vi "13-ATC예문.vi"() -> ()   [LabVIEW 2014]
doc: "ATC app"
uses:
  <vilib>/Utility/sysdir.llb/System Directory Type.ctl
panel:
  in  "정규식 3":string
  out "ip address":string="ip address 를 불러옵니다."
  in  "정규식":string
  in  "정규식 2":string
  out "연결된 문자열":string
  in  "탭 컨트롤":T1(tab)
  in  "메모":string="필요한 메모를 할수 있습니다. "
  in  "SID&RadarVector. 2":string="SID&RadarVector. "
  in  "인사말":string="인사말"
  in  "관제기관":string="관제기관"
  in  "콜사인":string="콜사인\n콜사인\n콜사인"
  in  "도착공항":string="도착공항"
  in  "SID&RadarVector":string="SID&RadarVector"
  in  "비행고도":string="비행고도"
  in  "인사말2":string="인사말"
  in  "콜사인2":string="콜사인"
  in  "콜사인3":string="콜사인"
  in  "콜사인4":string="콜사인"
  in  "콜사인5":string="콜사인"
  in  "콜사인6":string="콜사인"
  in  "도착공항2":string="도착공항"
  in  "제한고도":string="제한고도"
  in  "비행고도2":string="비행고도"
  in  "D접속주파수":string="접속주파수"
  in  "스콱번호":string="스콱번호"
  in  "도착공항3":string="도착공항"
  in  "SID&RadarVector. 3":string="SID&RadarVector. "
  in  "제한고도2":string="제한고도"
  in  "비행고도3":string="비행고도"
  in  "D접속주파수2":string="접속주파수"
  in  "스콱번호2":string="스쾃번호"
  in  "콜사인7":string="콜사인"
  in  "콜사인8":string="콜사인"
  in  "관제기관":string="관제기관"
  in  "G접속주파수2":string="접속주파수"
  in  "관제기관":string="관제기관"
  in  "G접속주파수":string="접속주파수"
  in  "콜사인9":string="콜사인"
  in  "정보1":bool
  in  "메모2":string="필요한 메모를 할수 있습니다. "
  in  "관제기관":string="관제기관"
  in  "콜사인24":string="콜사인"
  in  "T접속주파수2":string="접속주파수"
  in  "T접속주파수":string="접속주파수"
  in  "관제기관":string="관제기관"
  in  "콜사인23":string="콜사인"
  in  "활주로9":string="활주로"
  in  "관제기관":string="관제기관"
  in  "콜사인22":string="콜사인"
  in  "콜사인21":string="콜사인"
  in  "콜사인20":string="콜사인"
  in  "콜사인19":string="콜사인"
  in  "활주로8":string="활주로"
  in  "활주로7":string="활주로"
  in  "콜사인17":string="콜사인"
  in  "활주로6":string="활주로"
  in  "콜사인18":string="콜사인"
  in  "관제기관":string="관제기관"
  in  "then2":string="than"
  in  "활주로5":string="활주로"
  in  "콜사인16":string="콜사인"
  in  "then":string="than"
  in  "활주로4":string="활주로"
  in  "콜사인15":string="콜사인"
  in  "활주로3":string="활주로"
  in  "관제기관":string="관제기관"
  in  "콜사인14":string="콜사인"
  in  "콜사인13":string="콜사인"
  in  "현재기압2":string="현재기압"
  in  "출발공항":string="출발공항"
  in  "활주로2":string="활주로"
  in  "현재기압":string="현재기압"
  in  "출발공항":string="출발공항"
  in  "활주로1":string="활주로"
  in  "콜사인12":string="콜사인"
  in  "콜사인11":string="콜사인"
  in  "관제기관":string="관제기관"
  in  "인사3":string="인사"
  in  "정보2":bool
  in  "메모3":string="필요한 메모를 할수 있습니다. "
  in  "인사4":string="인사"
  in  "콜사인25":string="콜사인"
  in  "활주로10":string="활주로"
  in  "콜사인26":string="콜사인"
  in  "바람방향":string="바람방향"
  in  "풍속":string="풍속"
  in  "콜사인27":string="콜사인"
  in  "바람방향2":string="바람방향"
  in  "풍속2":string="풍속"
  in  "활주로11":string="활주로"
  in  "콜사인28":string="콜사인"
  in  "활주로13":string="활주로"
  in  "콜사인29":string="콜사인"
  in  "활주로12":string="활주로"
  in  "콜사인30":string="콜사인"
  in  "활주로14":string="활주로"
  in  "콜사인31":string="콜사인"
  in  "활주로15":string="활주로"
  in  "관제기관":string="관제기관"
  in  "콜사인32":string="콜사인"
  in  "현재고도":string="현재고도"
  in  "허가고도":string="허가고도"
  in  "콜사인33":string="콜사인"
  in  "접속주파수":string="접속주파수"
  in  "콜사인34":string="콜사인"
  in  "접속주파수2":string="접속주파수"
  in  "정보3":bool
  in  "메모 4":string="필요한 메모를 할수 있습니다. "
  in  "인사5":string="인사"
  in  "관제기관":string="관제기관"
  in  "콜사인35":string="콜사인"
  in  "거리":string="거리"
  in  "지점":string="지점"
  in  "현재고도A":string="현재고도"
  in  "허가고도3":string="허가고도"
  in  "콜사인36":string="콜사인"
  in  "관제기관":string="관제기관"
  in  "허가고도4":string="허가고도"
  in  "허가고도5":string="허가고도"
  in  "콜사인37":string="콜사인"
  in  "콜사인38":string="콜사인"
  in  "허가고도6":string="허가고도"
  in  "허가고도7":string="허가고도"
  in  "콜사인39":string="콜사인"
  in  "콜사인40":string="콜사인"
  in  "거리2":string="거리"
  in  "지점2":string="지점"
  in  "관제기관":string="관제기관"
  in  "A접속주파수":string="접속주파수"
  in  "관제기관":string="관제기관"
  in  "A접속주파수2":string="접속주파수"
  in  "콜사인41":string="콜사인"
  in  "정보4":bool
  in  "콜사인42":string="콜사인"
  in  "관제기관":string="관제기관"
  in  "A접속주파수":string="접속주파수"
  in  "콜사인45":string="콜사인"
  in  "관제기관":string="관제기관"
  in  "A접속주파수2":string="접속주파수"
  in  "관제기관":string="관제기관"
  in  "콜사인46":string="콜사인"
  in  "날시정보":string="날시정보"
  in  "고도":string="고도"
  in  "콜사인47":string="콜사인"
  in  "관제기관":string="관제기관"
  in  "L활주로":string="활주로"
  in  "도착공항4":string="도착공항"
  in  "현재기압":string="현재기압"
  in  "콜사인48":string="콜사인"
  in  "관제기관5":string="관제기관"
  in  "L활주로":string="활주로"
  in  "도착공항5":string="도착공항"
  in  "현재기압":string="현재기압"
  in  "콜사인49":string="콜사인"
  in  "고도":string="고도"
  in  "콜사인50":string="콜사인"
  in  "고도":string="고도"
  in  "콜사인51":string="콜사인"
  in  "고도":string="고도"
  in  "고도":string="고도"
  in  "콜사인52":string="콜사인"
  in  "콜사인53":string="콜사인"
  in  "관제기관":string="관제기관"
  in  "풍속":string="풍속"
  in  "바람방향":string="바람방향"
  in  "L활주로3":string="활주로"
  in  "콜사인54":string="콜사인"
  in  "풍속2":string="풍속"
  in  "바람방향2":string="바람방향"
  in  "L활주로":string="활주로"
  in  "콜사인55":string="콜사인"
  in  "관제기관":string="관제기관"
  in  "L활주로":string="활주로"
  in  "ILS":string="주파수(ils)"
  in  "콜사인56":string="콜사인"
  in  "L활주로6":string="활주로"
  in  "ILS2":string="주파수(ils)"
  in  "관제기관":string="관제기관"
  in  "콜사인57":string="콜사인"
  in  "T관제기관":string="관제기관"
  in  "T접속주파수":string="접속주파수"
  in  "콜사인58":string="콜사인"
  in  "콜사인59":string="콜사인"
  in  "관제기관":string="관제기관"
  in  "T접속주파수":string="접속주파수"
  in  "정보5":bool
  in  "메모5":string="필요한 메모를 할수 있습니다. "
  in  "바람방향":string="바람방향"
  in  "관제기관":string="관제기관"
  in  "콜사인60":string="콜사인"
  in  "L활주로7":string="활주로"
  in  "콜사인61":string="콜사인"
  in  "풍속":string="풍속"
  in  "콜사인62":string="콜사인"
  in  "L활주로":string="활주로"
  in  "L활주로":string="활주로"
  in  "관제기관":string="관제기관"
  in  "콜사인63":string="콜사인"
  in  "거리":string="거리"
  in  "관제기관3":string="관제기관"
  in  "콜사인64":string="콜사인"
  in  "L활주로":string="활주로"
  in  "G관제기관":string="관제기관"
  in  "G접속주파수":string="접속주파수"
  in  "콜사인65":string="콜사인"
  in  "관제기관":string="관제기관"
  in  "G접속주파수":string="접속주파수"
  in  "정보6":bool
  in  "메모 6":string="필요한 메모를 할수 있습니다. "
  in  "관제기관":string="관제기관"
  in  "콜사인66":string="콜사인"
  in  "콜사인67":string="콜사인"
  in  "게이트번호":string="게이트번호"
  in  "THEN":string="then"
  in  "콜사인68":string="콜사인"
  in  "게이트번호2":string="게이트번호"
  in  "THEN2":string="then"
  in  "관제기관2":string="관제기관"
  in  "콜사인69":string="콜사인"
  in  "C활주로":string="활주로"
  in  "관제기관3":string="관제기관"
  in  "C활주로2":string="활주로"
  in  "C활주로3":string="활주로"
  in  "콜사인70":string="콜사인"
  in  "콜사인10":string="콜사인"
  in  "관제기관4":string="관제기관"
  in  "콜사인71":string="콜사인"
  in  "콜사인72":string="콜사인"
  in  "정보7":bool
  # "ver.Beta.1.0.1"
  # "~"
  # "Good"
  # "Clearance Delivery"
  # "Pilot"
  # "at FL"
  # "Request Clearance IFR to"
  # "Airport via"
  # "~"
  # "Good"
  # "Controller"
  # ",  Clearance  Delivery, standby."
  # "Pilot"
  # "Stand by,"
  # "Controller"
  # ", Clearance  또는 Clearence, Are you ready to copy?"
  # "Pilot"
  # "Go Ahead 또는 Ready to copy"
  # "Airport via"
  # ", Cleared to"
  # "Controller"
  # "ft expect FL"
  # "then as filed. Climb and Maintain"
  # "Departure Frequency"
  # "Read back."
  # "Squawk"
  # "Pilot"
  # "Airport via"
  # "Cleared to"
  # ","
  # "then as filed."
  # "Climb and Maintain"
  # "ft expect FL"
  # "Departure Frequency"
  # "and we'll Squawk"
  # "Controller"
  # ", Read back is corrent contact"
  # "Ground"
  # "bye bye~."
  # "Pilot"
  # "Roger, contact"
  # ", bye bye~"
  # "ver.Beta.1.0.1"
  # "Pilot"
  # "~"
  # "Good"
  # "When ready for push back and Engine Start."
  # ","
  # "Request push back and Engine start and when ready to taxi to the Rwy"
  # "Controller"
  # ","
  # "QNH  Read Back."
  # "Pilot"
  # "Roger\nPush back and Engine start and when ready to taxi to the Rwy"
  # "Ready for taxi to the Rwy"
  # ","
  # "- Push back 완료 후 -"
  # "Ready for taxi to the Rwy"
  # ","
  # "Controller"
  # ", taxi to hold short of Rwy"
  # "via taxiway"
  # ", Roger"
  # "Pilot"
  # "via taxiway"
  # "Taxi to hold short of Rwy"
  # "- 활주로를 건널 상황일 때 -"
  # "Pilot"
  # "Request Cross Rwy"
  # ","
  # "Controller"
  # ", Cross Rwy"
  # "approved."
  # "Pilot"
  # "Cross Rwy"
  # "Approved"
  # "Controller"
  # ", Change squawk mode standby for mode 'C'"
  # "Pilot"
  # ", Roger Change squawk mode 'C'"
  # "------------------------ 홀딩 포인트 도착 후 ----------------------------------"
  # "hold short of Rwy"
  # ","
  # "Controller"
  # "Roger,"
  # "contact"
  # "Tower"
  # "bye bye~"
  # "Pilot"
  # "Contact"
  # "ver.Beta.1.0.1"
  # "Pilot"
  # "Good"
  # "~"
  # ",  hold short Rwy"
  # ", Ready for Departure"
  # "(곧바로 이륙허가)"
  # "Controller"
  # ", wind"
  # "knot, cleared for take off."
  # "at"
  # "Pilot"
  # "Knot, Clear for take off Rwy"
  # "Wind"
  # "at"
  # "Roger,"
  # "(활주로 정렬대기)"
  # "Controller"
  # ", Line up Rwy"
  # "(혹은 Taxi into position and Hold rwy"
  # ")"
  # "Pilot"
  # "또는  Taxi into position and Hold Rwy"
  # "Line up Rwy"
  # ")"
  # "Roger,"
  # "(홀딩 포인트에서 대기)"
  # "Controller"
  # ", Hold short rwy"
  # ","
  # "Pilot"
  # "Line up Rwy"
  # "Roger,"
  # "- 이 륙 후 -"
  # "Pilot"
  # "Airborn Passing"
  # "ft, Climbing"
  # ","
  # "ft."
  # "Controller"
  # ", contact Unicom Frequency"
  # "bye bye~"
  # "Pilot"
  # ", Roger"
  # "Contact Unicom Frequency"
  # "bye bye~"
  # "ver.Beta.1.0.1"
  # "Good"
  # "~"
  # "Pilot"
  # "Miles of"
  # "Intersection Passing FL"
  # ","
  # ","
  # "for FL"
  # "Controller"
  # "Center, Climb and Maintain"
  # ","
  # "."
  # "Pilot"
  # "Roger Climb and Maintain FL"
  # ","
  # "- 하 강 발 부 -"
  # "Controller"
  # "Decend and maintain FL"
  # "Pilot"
  # "Decend and maintain FL"
  # ","
  # "Controller"
  # "Approach"
  # "Mile from"
  # ". Contact"
  # ","
  # "Pilot"
  # "Contact"
  # "G'day"
  # "Approach"
  # ","
  # "Controller"
  # "ver.Beta.1.0.1"
  # "Approach"
  # ", Change"
  # "Pilot"
  # ", Roger"
  # "Change"
  # ","
  # "Pilot"
  # ","
  # "with you at FL"
  # "with information"
  # ","
  # ", Expect vector to ILS Rwy"
  # "final approach"
  # "Controller"
  # "QNH"
  # "Roger,"
  # "Pilot"
  # ", Expect vector to ILS Rwy"
  # "final approach"
  # "QNH"
  # "Controller"
  # ", Decend and maintain FL"
  # "Pilot"
  # "Decend and maintain FL"
  # "Roger,"
  # "Controller"
  # ", Decend and maintain"
  # "ft"
  # "Pilot"
  # "Roger"
  # "Decend and maintain"
  # "ft"
  # "Controller"
  # ","
  # "for landing"
  # "wind"
  # "knots active Rwy"
  # "at"
  # "Roger,"
  # "Pilot"
  # "Wind"
  # "knots active Rwy"
  # "for landing"
  # "at"
  # "Controller"
  # ","
  # "approach use Rwy"
  # "ILS"
  # "Roger,"
  # "Pilot"
  # "Use Rwy"
  # "ILS"
  # "- 정 렬 후 -"
  # "Pilot"
  # ","
  # "LOC and GS Capture"
  # "Controller"
  # "bye bye~"
  # "Roger, Contact"
  # "Pilot"
  # "Contact"
  # "Tower"
  # "G'Day~"
  # "ver.Beta.1.0.1"
  # "Pilot"
  # ","
  # "Inbound Approaching Rwy"
  # "Controller"
  # ", Wind"
  # "at"
  # "knots Rwy"
  # ", Cleared to land"
  # "Pilot"
  # "Rwy"
  # "Cleared to land"
  # "Pilot"
  # ","
  # "Miles"
  # "- 착 륙 후 -"
  # ","
  # "Pilot"
  # "Touch down with Rwy"
  # "Controller"
  # "Roger, change squawk mode Standby and contact"
  # "bye bye~"
  # "ground"
  # "Pilot"
  # ", Roger"
  # "bye bye~"
  # "Change squawk mode standby and contact"
  # "ver.Beta.1.0.1"
  # ","
  # "Pilot"
  # "Ready to taxi to the Gate"
  # "Controller"
  # ", taxi to the gate"
  # "via taxi way"
  # "Roger,"
  # "Pilot"
  # "taxi to the gate"
  # "via taxi way"
  # "- 활주로를 건널 상황일 때 -"
  # ","
  # "Request Cross Rwy"
  # "Controller"
  # ", Cross Rwy"
  # "approved."
  # "Pilot"
  # "Cross Rwy"
  # "approved"
  # "- 게이트 도착 후 -"
  # "Pilot"
  # "at Gate and Engine Shut down."
  # "Thank you for your ATC service."
  # "Controller"
  # ", at the gate and Engine Shut down, Thank you ~~"
  # "Pilot"
  # "Have a nice day,"
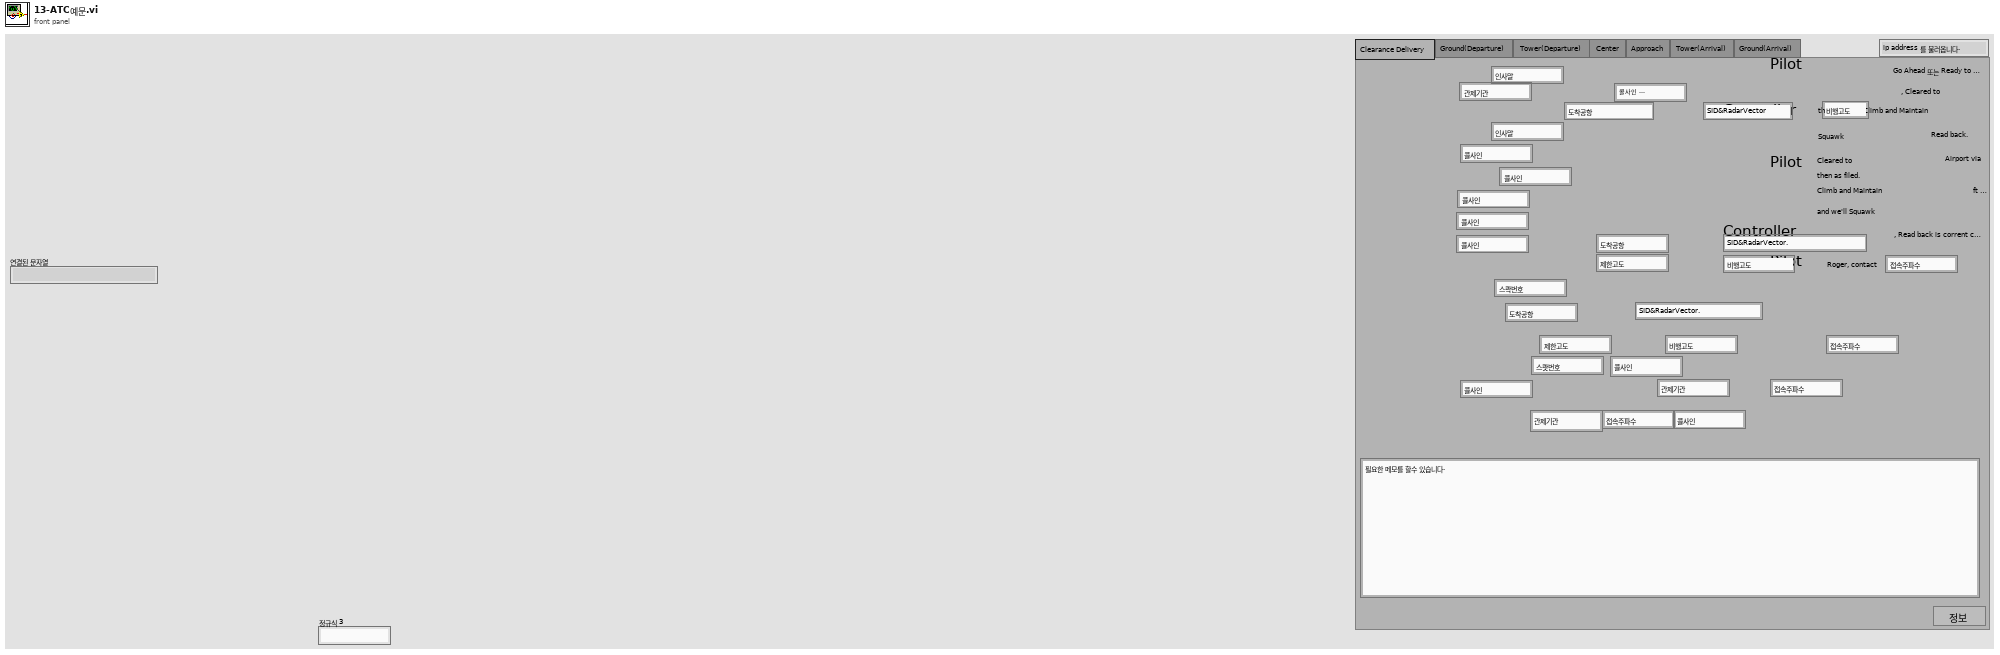
[diagram p1: front panel]
types:
  T1 = enum32{"Clearance Delivery", "Ground(Departure)", " Tower(Departure)", "Center ", "Approach", "Tower(Arrival) ", "Ground(Arrival)"}
  T2 = enum16{"open", "replace", "create", "open or create", "replace or create", "replace or create with confirmation"}
  T3 = typedef "System Directory Type.ctl" = i32
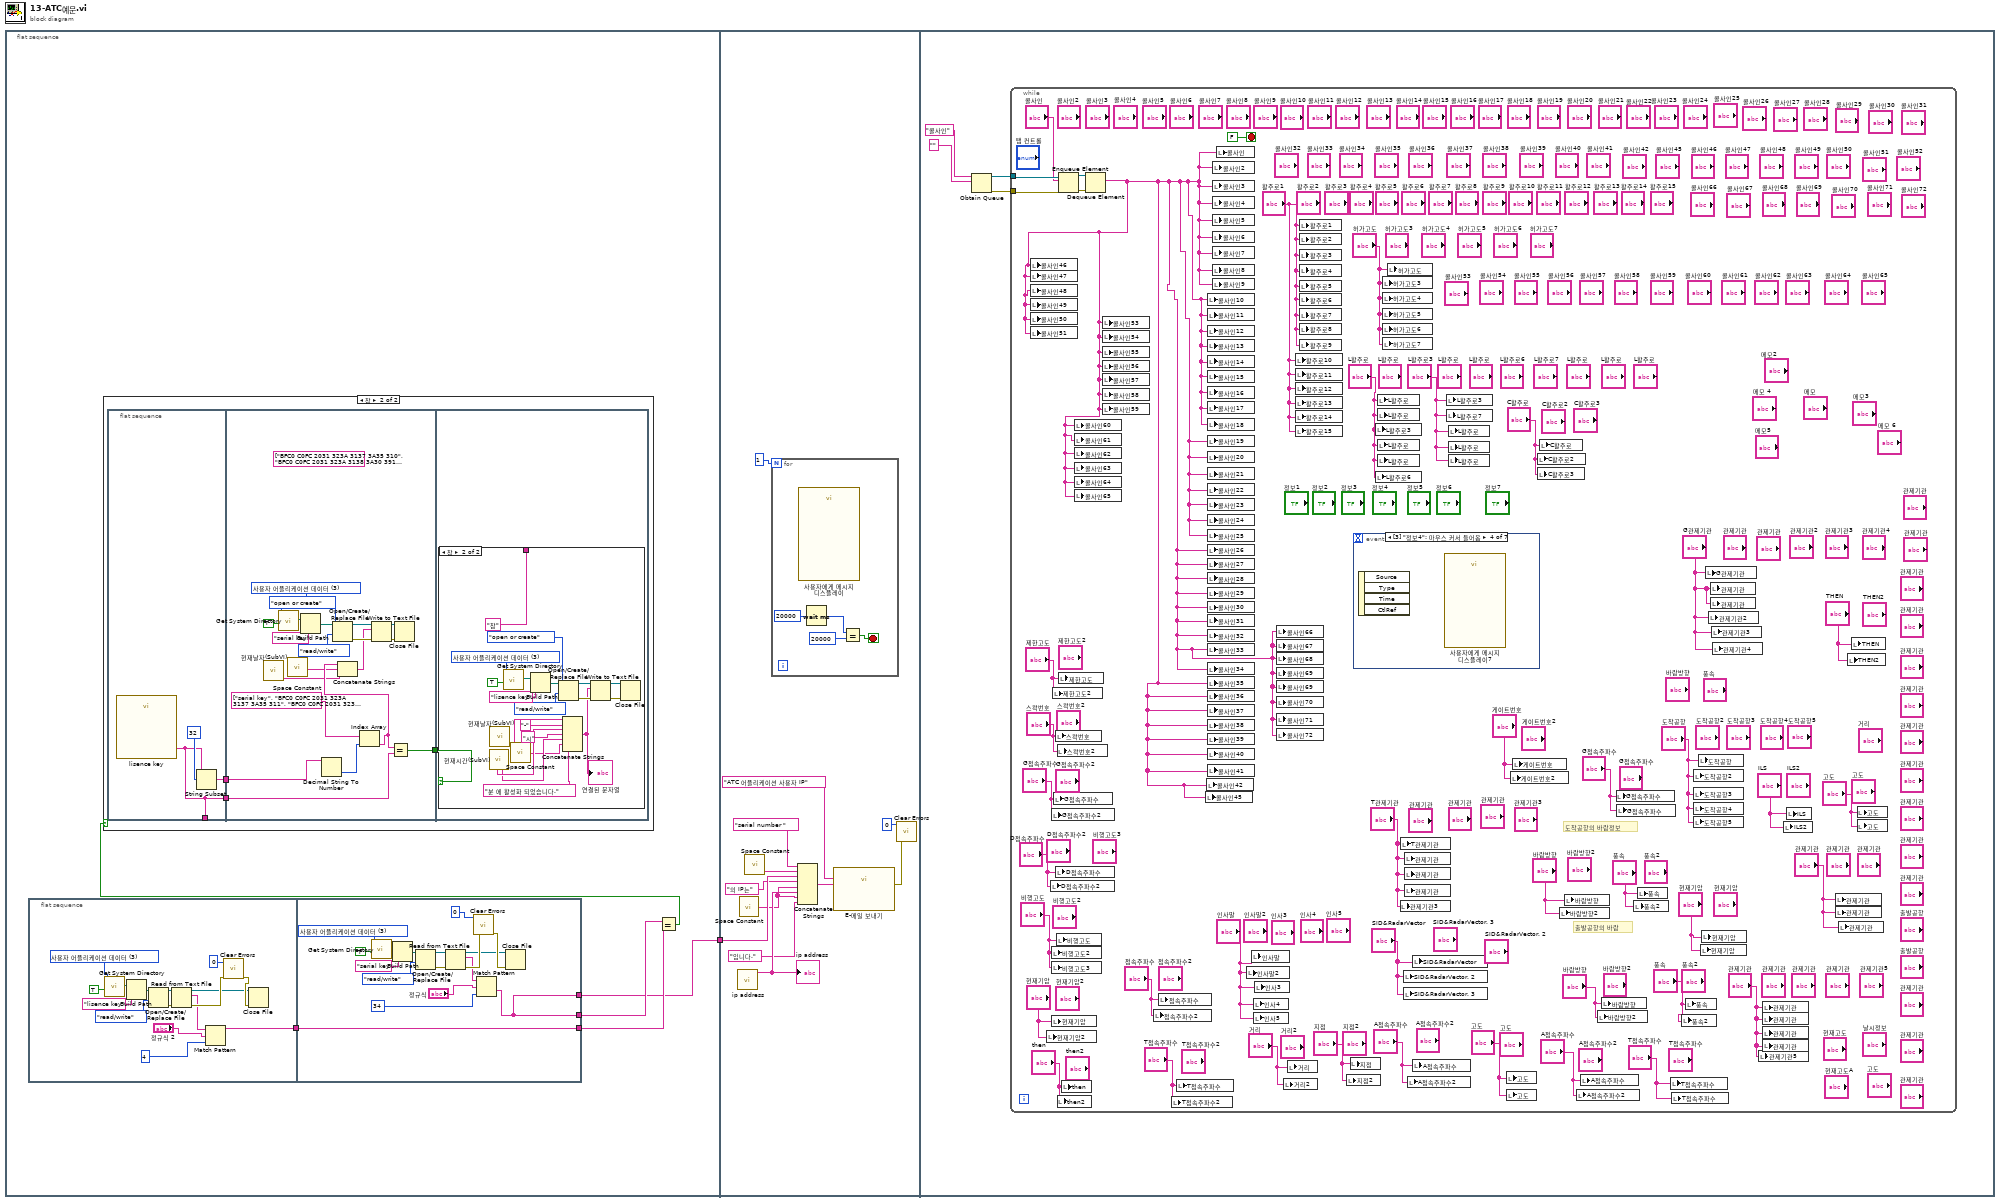
[diagram p0: block diagram]
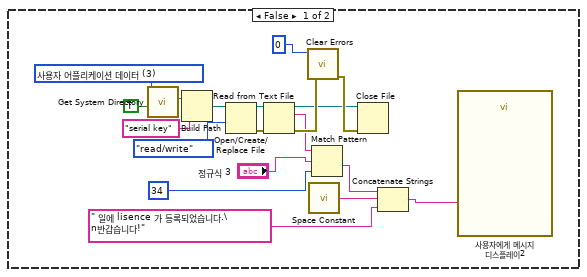
[diagram p2: hidden frame]
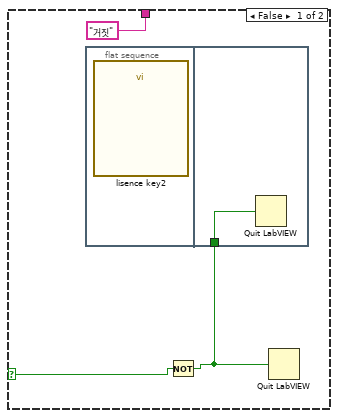
[diagram p3: hidden frame]
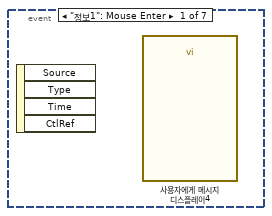
[diagram p4: hidden frame]
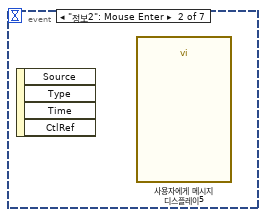
[diagram p5: hidden frame]
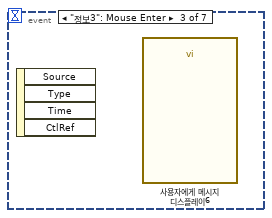
[diagram p6: hidden frame]
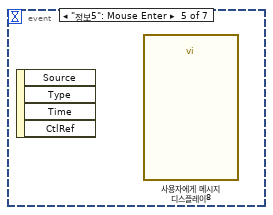
[diagram p7: hidden frame]
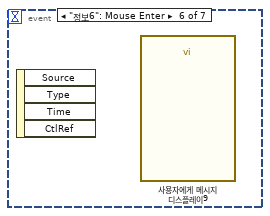
[diagram p8: hidden frame]
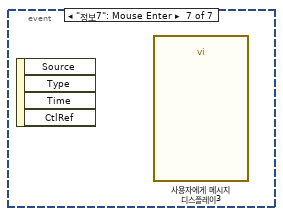
[diagram p9: hidden frame]
diagram:
  n1 = flat-sequence {
    tunnel: [w2] -> w1
    tunnel: w1 -> [w120]
    frame #0 {
      n2 = flat-sequence {
        tunnel: [w7] -> w6
        tunnel: [w26] -> w5
        tunnel: w6 -> [w26]
        tunnel: [w24] -> w4
        tunnel: [w24] -> w2
        frame #0 {
          w12 = T3 3 items=["사용자 홈"=0, "사용자 데스크탑"=1, "사용자 문서"=2, "사용자 어플리케이션 데이터"=3, "사용자 환경"=4, "사용자 임시"=5, "퍼블릭 문서"=6, "퍼블릭 어플리케이션 데이터"=7, "퍼블릭 환경"=8, "퍼블릭 캐시"=13, "시스템 코어 라이브러리"=9, "시스템 설치된 라이브러리"=10, "어플리케이션 파일"=11, "부팅 볼륨 루트"=12] ("system directory type")
          n3 = call <vilib>:"Get System Directory.vi"("create directory if not found? (F)"=TRUE, "system directory type"=w12) -> ("system directory"=w11:path)  [unwired: 9 in]
          n4 = Build Path(base path=w11, name or relative path="lisence key" ("이름 또는 상대 경로")) -> (appended path=w10:path)
          n5 = Open/Create/Replace File(file path (use dialog)=w10, access (0:read/write)=enum16{"read/write", "read-only", "write-only"}."read/write" ("접근(0:읽기/쓰기)")) -> (refnum out=w16:refnum<file>, error out=w15:errorcluster)  [unwired: 4 in, 1 out]
          n6 = Read from Text File(file (use dialog)=w16, error in=w15) -> (refnum out=w17:refnum<file>, text=w18:string, error out=w20:errorcluster)  [unwired: 2 in, 1 out]
          n7 = Match Pattern(string=w18, regular expression="정규식 2", offset (0)=4 ("오프셋(0) 2")) -> (before substring=w7:string)  [unwired: 3 out]
          n8 = call <vilib>:"Clear Errors.vi"("error in (no error)"=w20, "specific error code to clear (0: all)"=0) -> ("error out"=w21:errorcluster)  [unwired: 4 in, 1 out]
          n9 = Close File(refnum=w17, error in=w21) -> ()  [unwired: 2 out]
        }
        frame #1 {
          w32 = T3 3 items=["사용자 홈"=0, "사용자 데스크탑"=1, "사용자 문서"=2, "사용자 어플리케이션 데이터"=3, "사용자 환경"=4, "사용자 임시"=5, "퍼블릭 문서"=6, "퍼블릭 어플리케이션 데이터"=7, "퍼블릭 환경"=8, "퍼블릭 캐시"=13, "시스템 코어 라이브러리"=9, "시스템 설치된 라이브러리"=10, "어플리케이션 파일"=11, "부팅 볼륨 루트"=12] ("system directory type")
          n10 = call <vilib>:"Get System Directory.vi"("create directory if not found? (F)"=TRUE, "system directory type"=w32) -> ("system directory"=w33:path)  [unwired: 9 in]
          n11 = Build Path(base path=w33, name or relative path="serial key" ("이름 또는 상대 경로")) -> (appended path=w34:path)
          n12 = Open/Create/Replace File(file path (use dialog)=w34, access (0:read/write)=enum16{"read/write", "read-only", "write-only"}."read/write" ("접근(0:읽기/쓰기)")) -> (refnum out=w28:refnum<file>, error out=w29:errorcluster)  [unwired: 4 in, 1 out]
          n13 = Read from Text File(file (use dialog)=w28, error in=w29) -> (refnum out=w27:refnum<file>, text=w35:string, error out=w37:errorcluster)  [unwired: 2 in, 1 out]
          n14 = call <vilib>:"Clear Errors.vi"("error in (no error)"=w37, "specific error code to clear (0: all)"=0) -> ("error out"=w38:errorcluster)  [unwired: 4 in, 1 out]
          n15 = Match Pattern(string=w35, regular expression="정규식", offset (0)=34 ("오프셋(0)")) -> (after substring=w24:string)  [unwired: 3 out]
          n16 = Close File(refnum=w27, error in=w38) -> ()  [unwired: 2 out]
        }
      }
      n17 = Equal?(x=w4, y=w5) -> (x = y?=w3:bool)
      n18 = case shown="참" w3 {
        frame False {
          w52 = T3 3 items=["사용자 홈"=0, "사용자 데스크탑"=1, "사용자 문서"=2, "사용자 어플리케이션 데이터"=3, "사용자 환경"=4, "사용자 임시"=5, "퍼블릭 문서"=6, "퍼블릭 어플리케이션 데이터"=7, "퍼블릭 환경"=8, "퍼블릭 캐시"=13, "시스템 코어 라이브러리"=9, "시스템 설치된 라이브러리"=10, "어플리케이션 파일"=11, "부팅 볼륨 루트"=12] ("system directory type")
          n19 = call <vilib>:"Get System Directory.vi"("create directory if not found? (F)"=TRUE, "system directory type"=w52) -> ("system directory"=w53:path)  [unwired: 9 in]
          n20 = Build Path(base path=w53, name or relative path="serial key" ("이름 또는 상대 경로")) -> (appended path=w54:path)
          n21 = Open/Create/Replace File(file path (use dialog)=w54, access (0:read/write)=enum16{"read/write", "read-only", "write-only"}."read/write" ("접근(0:읽기/쓰기)")) -> (refnum out=w48:refnum<file>, error out=w49:errorcluster)  [unwired: 4 in, 1 out]
          n22 = Read from Text File(file (use dialog)=w48, error in=w49) -> (refnum out=w47:refnum<file>, text=w55:string, error out=w57:errorcluster)  [unwired: 2 in, 1 out]
          n23 = call <vilib>:"Clear Errors.vi"("error in (no error)"=w57, "specific error code to clear (0: all)"=0) -> ("error out"=w58:errorcluster)  [unwired: 4 in, 1 out]
          n24 = call <vilib>:"Space Constant.vi"() -> ("String"=w41:string)
          n25 = Match Pattern(string=w55, regular expression="정규식 3", offset (0)=34 ("오프셋(0)")) -> (after substring=w44:string)  [unwired: 3 out]
          n26 = Close File(refnum=w47, error in=w58) -> ()  [unwired: 2 out]
          n27 = Concatenate Strings(w44, w41, " 일에 lisence 가 등록되었습니다.\n반갑습니다!" ("Message")) -> (w43:string)
          n28 = call "사용자에게 메시지 디스플레이2"("Message"=w43) -> ()  [unwired: 9 in, 2 out]
        }
        frame True {
          n29 = flat-sequence {
            tunnel: [w63] -> w61
            tunnel: [w62] -> w60
            tunnel: [w62] -> _
            tunnel: w61 -> [w84]
            tunnel: [w81] -> w59
            tunnel: w60 -> [w82]
            tunnel: w59 -> [w85]
            frame #0 {
              n30 = call "lisence key"() -> ("lisence key"=w62:string)  [unwired: 17 in, 2 out]
              n31 = String Subset(string=w62, offset (0)=32 ("오프셋(0)")) -> (substring=w63:string)  [unwired: 1 in]
            }
            frame #1 {
              w74 = T3 3 items=["사용자 홈"=0, "사용자 데스크탑"=1, "사용자 문서"=2, "사용자 어플리케이션 데이터"=3, "사용자 환경"=4, "사용자 임시"=5, "퍼블릭 문서"=6, "퍼블릭 어플리케이션 데이터"=7, "퍼블릭 환경"=8, "퍼블릭 캐시"=13, "시스템 코어 라이브러리"=9, "시스템 설치된 라이브러리"=10, "어플리케이션 파일"=11, "부팅 볼륨 루트"=12] ("system directory type")
              (unwired) string[] ["BFC0 C0FC 2031 323A 3137 3A35 310", "BFC0 C0FC 2031 323A 3138 3A30 391", "BFC0 C0FC 2031 323A 3139 3A30 392", "BFC0 C0FC 2031 323A 3230 3A30 393", "BFC0 C0FC 2031 323A 3231 3A30 394", "BFC0 C0FC 2031 323A 3232 3A30 395", "BFC0 C0FC 2031 323A 3233 3A30 396", "BFC0 C0FC 2031 323A 3234 3A30 397", "BFC0 C0FC 2031 323A 3235 3A30 398", "BFC0 C0FC 2031 323A 3236 3A30 399", "BFC0 C0FC 2031 323A 3237 3A30 3910", "BFC0 C0FC 2031 323A 3238 3A30 3911", "BFC0 C0FC 2031 323A 3239 3A30 3912", "BFC0 C0FC 2031 323A 3036 3A33 3213", "BFC0 C0FC 2031 323A 3037 3A33 3214", "BFC0 C0FC 2031 323A 3038 3A33 3215", "BFC0 C0FC 2031 323A 3038 3A33 3216", "BFC0 C0FC 2031 323A 3039 3A33 3217", "BFC0 C0FC 2031 323A 3039 3A35 3018", "BFC0 C0FC 2031 323A 3130 3A35 3019", "BFC0 C0FC 2031 323A 3131 3A35 3120", "BFC0 C8C4 2031 313A 3536 3A33 3221", "BFC0 C8C4 2031 313A 3537 3A33 3222", "BFC0 C8C4 2031 313A 3538 3A33 3223", "BFC0 C8C4 2031 313A 3539 3A33 3224", "BFC0 C0FC 2031 323A 3030 3A33 3225", "BFC0 C0FC 2031 323A 3031 3A33 3226", "BFC0 C0FC 2031 323A 3032 3A33 3227", "BFC0 C0FC 2031 323A 3033 3A33 3228", "BFC0 C0FC 2031 323A 3034 3A33 3229", "BFC0 C0FC 2031 323A 3035 3A33 3230", "BFC0 C0FC 2031 323A 3036 3A33 3231", "BFC0 C0FC 2031 323A 3037 3A33 3232", "BFC0 C0FC 2031 323A 3038 3A33 3233"]
              n32 = call "현재날자(SubVI).vi"() -> ("월,일 을 문자열로"=w69:string)  [unwired: 5 in, 6 out]
              n33 = call <vilib>:"Get System Directory.vi"("create directory if not found? (F)"=TRUE, "system directory type"=w74) -> ("system directory"=w73:path)  [unwired: 9 in]
              n34 = call <vilib>:"Space Constant.vi"() -> ("String"=w68:string)
              n35 = Build Path(base path=w73, name or relative path="serial key" ("이름 또는 상대 경로")) -> (appended path=w72:path)
              n36 = Decimal String To Number(string=w84) -> (number=w83:i32)  [unwired: 2 in, 1 out]
              n37 = Open/Create/Replace File(file path (use dialog)=w72, operation (0:open)=T2."open or create" ("동작(0:open)"), access (0:read/write)=enum16{"read/write", "read-only", "write-only"}."read/write" ("접근(0:읽기/쓰기)")) -> (refnum out=w80:refnum<file>, error out=w79:errorcluster)  [unwired: 3 in, 1 out]
              n38 = Index Array(array=string[] ["serial key", "BFC0 C0FC 2031 323A 3137 3A35 311", "BFC0 C0FC 2031 323A 3138 3A30 392", "BFC0 C0FC 2031 323A 3139 3A30 393", "BFC0 C0FC 2031 323A 3230 3A30 394", "BFC0 C0FC 2031 323A 3231 3A30 395", "BFC0 C0FC 2031 323A 3232 3A30 396", "BFC0 C0FC 2031 323A 3233 3A30 397", "BFC0 C0FC 2031 323A 3234 3A30 398", "BFC0 C0FC 2031 323A 3235 3A30 399", "BFC0 C0FC 2031 323A 3236 3A30 3910", "BFC0 C0FC 2031 323A 3237 3A30 3911", "BFC0 C0FC 2031 323A 3238 3A30 3912", "BFC0 C0FC 2031 323A 3239 3A30 3913", "BFC0 C0FC 2031 323A 3036 3A33 3214", "BFC0 C0FC 2031 323A 3037 3A33 3215", "BFC0 C0FC 2031 323A 3038 3A33 3216", "BFC0 C0FC 2031 323A 3038 3A33 3217", "BFC0 C0FC 2031 323A 3039 3A33 3218", "BFC0 C0FC 2031 323A 3039 3A35 3019", "BFC0 C0FC 2031 323A 3130 3A35 3020", "BFC0 C0FC 2031 323A 3131 3A35 3121", "BFC0 C8C4 2031 313A 3536 3A33 3222", "BFC0 C8C4 2031 313A 3537 3A33 3223", "BFC0 C8C4 2031 313A 3538 3A33 3224", "BFC0 C8C4 2031 313A 3539 3A33 3225", "BFC0 C0FC 2031 323A 3030 3A33 3226", "BFC0 C0FC 2031 323A 3031 3A33 3227", "BFC0 C0FC 2031 323A 3032 3A33 3228", "BFC0 C0FC 2031 323A 3033 3A33 3229", "BFC0 C0FC 2031 323A 3034 3A33 3230", "BFC0 C0FC 2031 323A 3035 3A33 3231", "BFC0 C0FC 2031 323A 3036 3A33 3232", "BFC0 C0FC 2031 323A 3037 3A33 3233", "BFC0 C0FC 2031 323A 3038 3A33 3234", "BFC0 C0FC 2033 3A34 373A 3031 35 ", "BFC0 C0FC 2033 3A34 383A 3234 36", "BFC0 C0FC 2033 3A34 393A 3132 37", "BFC0 C0FC 2033 3A35 303A 3534 38", "BFC0 C0FC 2033 3A35 313A 3231 39 ", "BFC0 C0FC 2033 3A35 323A 3333 40 ", "BFC0 C0FC 2033 3A35 333A 3030 41", "BFC0 C0FC 2033 3A35 343A 3432 42", "BFC0 C0FC 2033 3A35 353A 3431 43", "BFC0 C0FC 2033 3A35 363A 3131 44", "BFC0 C0FC 2033 3A35 373A 3239 45", "BFC0 C0FC 2033 3A35 383A 3539 46", "BFC0 C0FC 2033 3A35 393A 3533 47", "BFC0 C0FC 2034 3A30 303A 3430 48 "] ("출력 배열"), index=w83) -> (element=w70:string)
              n39 = Concatenate Strings(w70, w68, w69) -> (w71:string)
              n40 = Write to Text File(file (use dialog)=w80, text=w71, error in=w79) -> (refnum out=w77:refnum<file>, error out=w78:errorcluster)  [unwired: 1 in, 1 out]
              n41 = Equal?(x=w70, y=w82) -> (x = y?=w81:bool)
              n42 = Close File(refnum=w77, error in=w78) -> ()  [unwired: 2 out]
            }
            frame #2 {
              n43 = case shown="참" w85 {
                selector: w85 -> [w86 _]
                tunnel: ["거짓" "참"] -> _
                frame False {
                  n44 = flat-sequence {
                    tunnel: w87 -> [w89]
                    frame #0 {
                      n45 = call "lisence key2"() -> ()  [unwired: 10 in, 2 out]
                    }
                    frame #1 {
                      n46 = Quit LabVIEW(quit? (T)=w89) -> ()
                    }
                  }
                  n47 = Not(x=w86) -> (.not. x?=w87:bool)
                  n48 = Quit LabVIEW(quit? (T)=w87) -> ()
                }
                frame True {
                  w105 = T3 3 items=["사용자 홈"=0, "사용자 데스크탑"=1, "사용자 문서"=2, "사용자 어플리케이션 데이터"=3, "사용자 환경"=4, "사용자 임시"=5, "퍼블릭 문서"=6, "퍼블릭 어플리케이션 데이터"=7, "퍼블릭 환경"=8, "퍼블릭 캐시"=13, "시스템 코어 라이브러리"=9, "시스템 설치된 라이브러리"=10, "어플리케이션 파일"=11, "부팅 볼륨 루트"=12] ("system directory type")
                  n49 = call "현재시간(SubVI).vi"() -> ("분 문자열"=w94:string, "시 문자열"=w96:string)  [unwired: 3 in, 7 out]
                  n50 = call "현재날자(SubVI).vi"() -> ("월,일 을 문자열로"=w98:string)  [unwired: 5 in, 6 out]
                  n51 = call <vilib>:"Get System Directory.vi"("create directory if not found? (F)"=TRUE, "system directory type"=w105) -> ("system directory"=w106:path)  [unwired: 9 in]
                  n52 = call <vilib>:"Space Constant.vi"() -> ("String"=w93:string)
                  n53 = Build Path(base path=w106, name or relative path="lisence key" ("이름 또는 상대 경로")) -> (appended path=w107:path)
                  n54 = Open/Create/Replace File(file path (use dialog)=w107, operation (0:open)=T2."open or create" ("동작(0:open)"), access (0:read/write)=enum16{"read/write", "read-only", "write-only"}."read/write" ("접근(0:읽기/쓰기)")) -> (refnum out=w103:refnum<file>, error out=w101:errorcluster)  [unwired: 3 in, 1 out]
                  n55 = Concatenate Strings(w98, "-", w96, "시", w94, w93, "분 에 활성화 되었습니다.") -> (w99:string)
                  "연결된 문자열" <- w99
                  n56 = Write to Text File(file (use dialog)=w103, text=w99, error in=w101) -> (refnum out=w104:refnum<file>, error out=w100:errorcluster)  [unwired: 1 in, 1 out]
                  n57 = Close File(refnum=w104, error in=w100) -> ()  [unwired: 2 out]
                }
              }
            }
          }
        }
      }
    }
    frame #1 {
      n58 = call "ip address.vi"() -> ("ip address"=w116:string)  [unwired: 11 in]
      "ip address" <- w116
      n59 = call <vilib>:"Space Constant.vi"() -> ("String"=w115:string)
      n60 = call <vilib>:"Space Constant.vi"() -> ("String"=w118:string)
      n61 = for {
        N: 1 -> [_]
        stop <- w124 stop-if-true
        n62 = call "사용자에게 메시지 디스플레이"() -> ()  [unwired: 10 in, 2 out]
        n63 = Wait (ms)(milliseconds to wait=u32 20000 ("대기 시간(ms)")) -> (millisecond timer value=w123:u32)
        n64 = Equal?(x=w123, y=u32 20000) -> (x = y?=w124:bool)
      }
      n65 = Concatenate Strings("serial number ", w118, w120, "의 IP는", w115, w116, w115, "입니다.") -> (w113:string)
      n66 = call "E-메일 보내기"("Message"=w113, "Subject"="ATC 어플리케이션 사용자 IP") -> ("error out"=w111:errorcluster)  [unwired: 9 in]
      n67 = call <vilib>:"Clear Errors.vi"("error in (no error)"=w111, "specific error code to clear (0: all)"=0) -> ()  [unwired: 4 in, 2 out]
    }
    frame #2 {
      n68 = Obtain Queue(name (unnamed)="콜사인", element data type="") -> (queue out=w129:refnum<queue>, error out=w128:errorcluster)  [unwired: 3 in, 1 out]
      n69 = while {
        tunnel: w129 -> [w172]
        tunnel: w128 -> [w171]
        stop <- FALSE stop-if-true
        # "도착공항의 바람정보"
        # "출발공항의 바람"
        n70 = local write "현재기압2"("현재기압") -> ()
        n71 = local write "D접속주파수2"("D접속주파수") -> ()
        n72 = local write "현재기압"("현재기압") -> ()
        n73 = local write "G접속주파수2"("G접속주파수") -> ()
        n74 = local write "비행고도2"("비행고도") -> ()
        n75 = local write "비행고도3"("비행고도") -> ()
        n76 = local write "제한고도2"("제한고도") -> ()
        n77 = local write "G접속주파수"("G접속주파수") -> ()
        n78 = local write "D접속주파수"("D접속주파수") -> ()
        n79 = local write "스콱번호"("스콱번호") -> ()
        n80 = local write "비행고도"("비행고도") -> ()
        n81 = local write "스콱번호2"("스콱번호") -> ()
        n82 = local write "then2"("then") -> ()
        n83 = Enqueue Element(queue=w172, element="콜사인", error in (no error)=w171) -> (queue out=w170:refnum<queue>, error out=w169:errorcluster)  [unwired: 1 in, 1 out]
        n84 = local write "제한고도"("제한고도") -> ()
        n85 = local write "then"("then") -> ()
        n86 = Dequeue Element(queue=w170, error in (no error)=w169) -> (element=w130:string)  [unwired: 1 in, 3 out]
        n87 = local write "콜사인46"(w130) -> ()
        n88 = local write "콜사인47"(w130) -> ()
        n89 = local write "콜사인48"(w130) -> ()
        n90 = local write "콜사인49"(w130) -> ()
        n91 = local write "콜사인50"(w130) -> ()
        n92 = local write "콜사인51"(w130) -> ()
        n93 = local write "콜사인60"(w130) -> ()
        n94 = local write "콜사인61"(w130) -> ()
        n95 = local write "콜사인62"(w130) -> ()
        n96 = local write "콜사인63"(w130) -> ()
        n97 = local write "콜사인64"(w130) -> ()
        n98 = local write "콜사인65"(w130) -> ()
        n99 = local write "콜사인53"(w130) -> ()
        n100 = local write "콜사인54"(w130) -> ()
        n101 = local write "콜사인55"(w130) -> ()
        n102 = local write "콜사인56"(w130) -> ()
        n103 = local write "콜사인57"(w130) -> ()
        n104 = local write "콜사인58"(w130) -> ()
        n105 = local write "콜사인59"(w130) -> ()
        n106 = local write "접속주파수2"("접속주파수") -> ()
        n107 = local write "접속주파수"("접속주파수") -> ()
        n108 = local write "T접속주파수2"("T접속주파수") -> ()
        n109 = local write "T접속주파수"("T접속주파수") -> ()
        n110 = local write "콜사인45"(w130) -> ()
        n111 = local write "콜사인42"(w130) -> ()
        n112 = local write "콜사인10"(w130) -> ()
        n113 = local write "콜사인11"(w130) -> ()
        n114 = local write "콜사인12"(w130) -> ()
        n115 = local write "콜사인13"(w130) -> ()
        n116 = local write "콜사인14"(w130) -> ()
        n117 = local write "콜사인15"(w130) -> ()
        n118 = local write "콜사인16"(w130) -> ()
        n119 = local write "콜사인17"(w130) -> ()
        n120 = local write "콜사인18"(w130) -> ()
        n121 = local write "콜사인19"(w130) -> ()
        n122 = local write "콜사인20"(w130) -> ()
        n123 = local write "콜사인21"(w130) -> ()
        n124 = local write "콜사인22"(w130) -> ()
        n125 = local write "콜사인23"(w130) -> ()
        n126 = local write "콜사인24"(w130) -> ()
        n127 = local write "콜사인25"(w130) -> ()
        n128 = local write "콜사인26"(w130) -> ()
        n129 = local write "콜사인27"(w130) -> ()
        n130 = local write "콜사인28"(w130) -> ()
        n131 = local write "콜사인29"(w130) -> ()
        n132 = local write "콜사인30"(w130) -> ()
        n133 = local write "콜사인31"(w130) -> ()
        n134 = local write "콜사인32"(w130) -> ()
        n135 = local write "콜사인33"(w130) -> ()
        n136 = local write "콜사인34"(w130) -> ()
        n137 = local write "콜사인35"(w130) -> ()
        n138 = local write "콜사인36"(w130) -> ()
        n139 = local write "콜사인37"(w130) -> ()
        n140 = local write "콜사인38"(w130) -> ()
        n141 = local write "콜사인39"(w130) -> ()
        n142 = local write "콜사인40"(w130) -> ()
        n143 = local write "콜사인41"(w130) -> ()
        n144 = local write "콜사인2"(w130) -> ()
        n145 = local write "콜사인3"(w130) -> ()
        n146 = local write "콜사인4"(w130) -> ()
        n147 = local write "콜사인5"(w130) -> ()
        n148 = local write "콜사인6"(w130) -> ()
        n149 = local write "콜사인7"(w130) -> ()
        n150 = local write "콜사인8"(w130) -> ()
        n151 = local write "콜사인9"(w130) -> ()
        n152 = local write "콜사인"(w130) -> ()
        n153 = local write "인사말2"("인사말") -> ()
        n154 = local write "인사말"("인사말") -> ()
        n155 = local write "인사4"("인사말") -> ()
        n156 = local write "인사5"("인사말") -> ()
        n157 = local write "인사3"("인사말") -> ()
        n158 = local write "콜사인66"(w130) -> ()
        n159 = local write "콜사인67"(w130) -> ()
        n160 = local write "콜사인68"(w130) -> ()
        n161 = local write "콜사인69"(w130) -> ()
        n162 = local write "콜사인69"(w130) -> ()
        n163 = local write "콜사인70"(w130) -> ()
        n164 = local write "콜사인71"(w130) -> ()
        n165 = local write "콜사인72"(w130) -> ()
        n166 = local write "거리2"("거리") -> ()
        n167 = local write "거리"("거리") -> ()
        n168 = local write "활주로10"("활주로1") -> ()
        n169 = local write "활주로11"("활주로1") -> ()
        n170 = local write "활주로12"("활주로1") -> ()
        n171 = local write "활주로13"("활주로1") -> ()
        n172 = local write "활주로14"("활주로1") -> ()
        n173 = local write "활주로15"("활주로1") -> ()
        n174 = local write "활주로1"("활주로1") -> ()
        n175 = local write "활주로2"("활주로1") -> ()
        n176 = local write "활주로3"("활주로1") -> ()
        n177 = local write "활주로4"("활주로1") -> ()
        n178 = local write "활주로5"("활주로1") -> ()
        n179 = local write "활주로6"("활주로1") -> ()
        n180 = local write "활주로7"("활주로1") -> ()
        n181 = local write "활주로8"("활주로1") -> ()
        n182 = local write "활주로9"("활주로1") -> ()
        n183 = local write "지점2"("지점") -> ()
        n184 = local write "지점"("지점") -> ()
        n185 = event shown="[3] \"정보4\": 마우스 커서 들어옴" {
          selector: _ -> [_ _ _ _ _ _ _]
          dyn-events: _ -> [_ _ _ _ _ _ _]
          timeout: _ -> [_ _ _ _ _ _ _]
          event "정보1": Mouse Enter {
            n186 = event-data() -> ()  [unwired: 1 in, 4 out]
            n187 = call "사용자에게 메시지 디스플레이4"() -> ()  [unwired: 10 in, 2 out]
          }
          event "정보2": Mouse Enter {
            n188 = event-data() -> ()  [unwired: 1 in, 4 out]
            n189 = call "사용자에게 메시지 디스플레이5"() -> ()  [unwired: 10 in, 2 out]
          }
          event "정보3": Mouse Enter {
            n190 = event-data() -> ()  [unwired: 1 in, 4 out]
            n191 = call "사용자에게 메시지 디스플레이6"() -> ()  [unwired: 10 in, 2 out]
          }
          event "정보4": Mouse Enter {
            n192 = event-data() -> ()  [unwired: 1 in, 4 out]
            n193 = call "사용자에게 메시지 디스플레이7"() -> ()  [unwired: 10 in, 2 out]
          }
          event "정보5": Mouse Enter {
            n194 = event-data() -> ()  [unwired: 1 in, 4 out]
            n195 = call "사용자에게 메시지 디스플레이8"() -> ()  [unwired: 10 in, 2 out]
          }
          event "정보6": Mouse Enter {
            n196 = event-data() -> ()  [unwired: 1 in, 4 out]
            n197 = call "사용자에게 메시지 디스플레이9"() -> ()  [unwired: 10 in, 2 out]
          }
          event "정보7": Mouse Enter {
            n198 = event-data() -> ()  [unwired: 1 in, 4 out]
            n199 = call "사용자에게 메시지 디스플레이3"() -> ()  [unwired: 10 in, 2 out]
          }
        }
        n200 = local write "L활주로3"("L활주로") -> ()
        n201 = local write "L활주로6"("L활주로") -> ()
        n202 = local write "L활주로"("L활주로") -> ()
        n203 = local write "L활주로"("L활주로") -> ()
        n204 = local write "L활주로"("L활주로") -> ()
        n205 = local write "L활주로"("L활주로") -> ()
        n206 = local write "허가고도3"("허가고도") -> ()
        n207 = local write "허가고도4"("허가고도") -> ()
        n208 = local write "허가고도5"("허가고도") -> ()
        n209 = local write "허가고도6"("허가고도") -> ()
        n210 = local write "허가고도7"("허가고도") -> ()
        n211 = local write "허가고도"("허가고도") -> ()
        n212 = local write "관제기관3"("T관제기관") -> ()
        n213 = local write "T관제기관"("T관제기관") -> ()
        n214 = local write "SID&RadarVector. 2"("SID&RadarVector") -> ()
        n215 = local write "SID&RadarVector. 3"("SID&RadarVector") -> ()
        n216 = local write "관제기관"("T관제기관") -> ()
        n217 = local write "관제기관"("T관제기관") -> ()
        n218 = local write "관제기관"("T관제기관") -> ()
        n219 = local write "A접속주파수2"("A접속주파수") -> ()
        n220 = local write "A접속주파수"("A접속주파수") -> ()
        n221 = local write "SID&RadarVector"("SID&RadarVector") -> ()
        n222 = local write "L활주로3"("L활주로3") -> ()
        n223 = local write "L활주로7"("L활주로3") -> ()
        n224 = local write "L활주로"("L활주로3") -> ()
        n225 = local write "L활주로"("L활주로3") -> ()
        n226 = local write "L활주로"("L활주로3") -> ()
        n227 = local write "고도"("고도") -> ()
        n228 = local write "고도"("고도") -> ()
        n229 = local write "게이트번호2"("게이트번호") -> ()
        n230 = local write "게이트번호"("게이트번호") -> ()
        n231 = local write "C활주로3"("C활주로") -> ()
        n232 = local write "C활주로2"("C활주로") -> ()
        n233 = local write "C활주로"("C활주로") -> ()
        n234 = local write "바람방향2"("바람방향") -> ()
        n235 = local write "바람방향"("바람방향") -> ()
        n236 = local write "A접속주파수2"("A접속주파수") -> ()
        n237 = local write "A접속주파수"("A접속주파수") -> ()
        n238 = local write "바람방향2"("바람방향") -> ()
        n239 = local write "바람방향"("바람방향") -> ()
        n240 = local write "G접속주파수"("G접속주파수") -> ()
        n241 = local write "G접속주파수"("G접속주파수") -> ()
        n242 = local write "풍속2"("풍속") -> ()
        n243 = local write "풍속"("풍속") -> ()
        n244 = local write "T접속주파수"("T접속주파수") -> ()
        n245 = local write "T접속주파수"("T접속주파수") -> ()
        n246 = local write "풍속2"("풍속") -> ()
        n247 = local write "풍속"("풍속") -> ()
        n248 = local write "도착공항2"("도착공항") -> ()
        n249 = local write "도착공항3"("도착공항") -> ()
        n250 = local write "도착공항4"("도착공항") -> ()
        n251 = local write "도착공항5"("도착공항") -> ()
        n252 = local write "도착공항"("도착공항") -> ()
        n253 = local write "현재기압"("현재기압") -> ()
        n254 = local write "현재기압"("현재기압") -> ()
        n255 = local write "G관제기관"("G관제기관") -> ()
        n256 = local write "관제기관2"("G관제기관") -> ()
        n257 = local write "관제기관"("G관제기관") -> ()
        n258 = local write "관제기관"("G관제기관") -> ()
        n259 = local write "관제기관3"("G관제기관") -> ()
        n260 = local write "관제기관4"("G관제기관") -> ()
        n261 = local write "관제기관5"("관제기관") -> ()
        n262 = local write "관제기관"("관제기관") -> ()
        n263 = local write "관제기관"("관제기관") -> ()
        n264 = local write "관제기관"("관제기관") -> ()
        n265 = local write "관제기관"("관제기관") -> ()
        n266 = local write "ILS2"("ILS") -> ()
        n267 = local write "ILS"("ILS") -> ()
        n268 = local write "관제기관"("관제기관") -> ()
        n269 = local write "관제기관"("관제기관") -> ()
        n270 = local write "관제기관"("관제기관") -> ()
        n271 = local write "THEN2"("THEN") -> ()
        n272 = local write "THEN"("THEN") -> ()
        n273 = local write "고도"("고도") -> ()
        n274 = local write "고도"("고도") -> ()
      }
    }
  }
